vi "Waveform Laser Control.vi"   [LabVIEW 2014]
uses:
  <vilib>/rvi/interface/nirviOpenFPGA/nirviOpenFPGA.xnode
  FPGA Bitfiles/MainSTEDFPGAProj_FPGATarget_WaveformandLaser_r4jCxZ5mzM0.lvbitx
  FPGA Target VIs/FPGA-7841R/Waveform and Laser Controls V3.vi
  <vilib>/FPGAPlugInAG/PCIe-7841R/niLvFpga_Open_PCIe-7841R.vi
  <vilib>/rvi/interface/common/dynamic/niFpgaDynamicAddResources.vi
  <vilib>/rvi/interface/nirviReadWriteControl/nirviReadWriteControl.xnode
  NiFpgaLv.dll
  <vilib>/Utility/error.llb/Error Cluster From Error Code.vi
  <vilib>/rvi/interface/Simulation/niFpgaSimulationCallBeginRW.vi
  <vilib>/rvi/errors/niLvFpgaAdjustHostInterfaceError.vi
  <vilib>/rvi/interface/nirviMethod/nirviMethod.xnode
  <vilib>/FPGAPlugInAG/Dynamic/niLvFpga_Run_Dynamic.vi
types:
  T1 = cluster{"Scanning Mode":u8, "Fast Axis WF Length (Elements)":i32, "Fast Axis Sample Period (Ticks)":u32, "Slow Axis 1 WF Length (Elements)":i32, "Slow Axis 1 Sample Period (Ticks)":u32, "Slow Axis 1 Delay (25 ns) Steps":i32, "Slow Axis 2 WFLength (Elements)":i32, "Slow Axis 2 Sample Period (Ticks)":u32, "Slow Axis 2 Delay (25 ns) Steps":i32}
  T2 = cluster{"Res Mirror Amp (I16)":i16, "Res Mirror Mute":bool}
  T3 = cluster{"AOM (Pin 51 AO4)":i16, "Beam Blanking":bool}
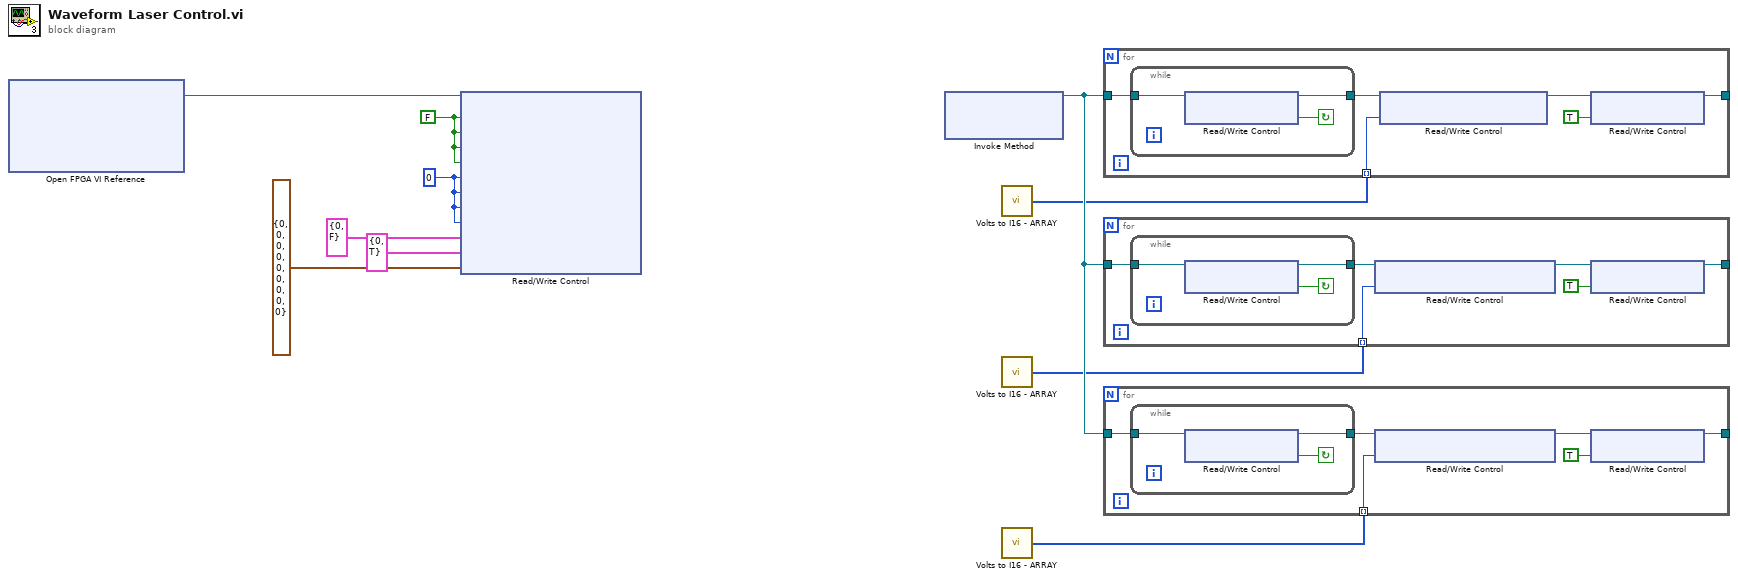
[diagram p0: block diagram]
diagram:
  w5 = i16 0 ("Fast Axis Waveform Element")
  w4 = FALSE ("WF 1 Data Loaded")
  n1 = xnode "Open FPGA VI Reference"() -> ("FPGA VI Reference Out"=w6:refnum<k20>)  [unwired: 2 in, 1 out]
  n2 = xnode "Read/Write Control"("FPGA VI Reference In"=w6, "WF 1 Data Loaded"=w4, "WF 2 Data Loaded"=w4, "WF 3 Data Loaded"=w4, "Start Waveforms"=w4, "Fast Axis Waveform Element"=w5, "Slow Axis 1 Waveform Element"=w5, "Slow Axis 2 Waveform Element"=w5, "Unused Axis Offset"=w5, "775 AOM"=T3 {"AOM (Pin 51 AO4)"=0, "Beam Blanking"=FALSE}, "Resoance Mirror"=T2 {"Res Mirror Amp (I16)"=0, "Res Mirror Mute"=TRUE}, "Waveform Scan Parameters"=T1 {"Scanning Mode"=0, "Fast Axis WF Length (Elements)"=0, "Fast Axis Sample Period (Ticks)"=0, "Slow Axis 1 WF Length (Elements)"=0, "Slow Axis 1 Sample Period (Ticks)"=0, "Slow Axis 1 Delay (25 ns) Steps"=0, "Slow Axis 2 WFLength (Elements)"=0, "Slow Axis 2 Sample Period (Ticks)"=0, "Slow Axis 2 Delay (25 ns) Steps"=0}) -> ()  [unwired: 1 in, 2 out]
  n3 = xnode "Invoke Method"() -> ("FPGA VI Reference Out"=w10:refnum<k20>)  [unwired: 3 in, 1 out]
  n4 = call "Volts to I16 - ARRAY.vi"() -> ("I16"=w9:i16[])  [unwired: 15 in]
  n5 = call "Volts to I16 - ARRAY.vi"() -> ("I16"=w8:i16[])  [unwired: 15 in]
  n6 = call "Volts to I16 - ARRAY.vi"() -> ("I16"=w7:i16[])  [unwired: 15 in]
  n7 = for {
    tunnel: w10 -> [w15]
    tunnel: [w13] -> _
    tunnel: w9 -> [w11] mode=indexing
    n8 = while {
      tunnel: w15 -> [w19]
      tunnel: [w18] -> w14
      stop <- w17 continue-if-true
      n9 = xnode "Read/Write Control"("FPGA VI Reference In"=w19) -> ("FPGA VI Reference Out"=w18:refnum<k20>, "WF 1 Data Loaded"=w17:bool)  [unwired: 1 in, 1 out]
    }
    n10 = xnode "Read/Write Control"("FPGA VI Reference In"=w14, "Fast Axis Waveform Element"=w11) -> ("FPGA VI Reference Out"=w16:refnum<k20>)  [unwired: 1 in, 1 out]
    n11 = xnode "Read/Write Control"("FPGA VI Reference In"=w16, "WF 1 Data Loaded"=TRUE ("Host Data Loaded")) -> ("FPGA VI Reference Out"=w13:refnum<k20>)  [unwired: 1 in, 1 out]
  }
  n12 = for {
    tunnel: w10 -> [w24]
    tunnel: [w22] -> _
    tunnel: w8 -> [w20] mode=indexing
    n13 = while {
      tunnel: w24 -> [w28]
      tunnel: [w27] -> w23
      stop <- w26 continue-if-true
      n14 = xnode "Read/Write Control"("FPGA VI Reference In"=w28) -> ("FPGA VI Reference Out"=w27:refnum<k20>, "WF 2 Data Loaded"=w26:bool)  [unwired: 1 in, 1 out]
    }
    n15 = xnode "Read/Write Control"("FPGA VI Reference In"=w23, "Slow Axis 1 Waveform Element"=w20) -> ("FPGA VI Reference Out"=w25:refnum<k20>)  [unwired: 1 in, 1 out]
    n16 = xnode "Read/Write Control"("FPGA VI Reference In"=w25, "WF 2 Data Loaded"=TRUE ("Host Data Loaded")) -> ("FPGA VI Reference Out"=w22:refnum<k20>)  [unwired: 1 in, 1 out]
  }
  n17 = for {
    tunnel: w10 -> [w33]
    tunnel: [w31] -> _
    tunnel: w7 -> [w29] mode=indexing
    n18 = while {
      tunnel: w33 -> [w37]
      tunnel: [w36] -> w32
      stop <- w35 continue-if-true
      n19 = xnode "Read/Write Control"("FPGA VI Reference In"=w37) -> ("FPGA VI Reference Out"=w36:refnum<k20>, "WF 3 Data Loaded"=w35:bool)  [unwired: 1 in, 1 out]
    }
    n20 = xnode "Read/Write Control"("FPGA VI Reference In"=w32, "Slow Axis 2 Waveform Element"=w29) -> ("FPGA VI Reference Out"=w34:refnum<k20>)  [unwired: 1 in, 1 out]
    n21 = xnode "Read/Write Control"("FPGA VI Reference In"=w34, "WF 3 Data Loaded"=TRUE ("Host Data Loaded")) -> ("FPGA VI Reference Out"=w31:refnum<k20>)  [unwired: 1 in, 1 out]
  }
